vi "Source and Sink Current.vi"(0 "Semiconductor Module Context":T1, 2 "Current level":dbl=0.001 caption="current level" format="%_6p", 5 "Pins":string[](array[string]), 11 "error in (no error)":errorcluster) -> (4 "Semiconductor Module Context Out":T1, 6 "Source Current measurements":dbl[](array[numeric]), 8 "Sink Current measurements":dbl[](array[numeric]), 15 "error out":errorcluster)   [LabVIEW 2013]
uses:
  <vilib>/NI_TestStand_SemiconductorModule/NI_TestStand_Semiconductor_Module.lvlibp/PinMap/General/SemiconductorModuleContext.ctl
  <vilib>/NI_TestStand_SemiconductorModule/NI_TestStand_Semiconductor_Module.lvlibp
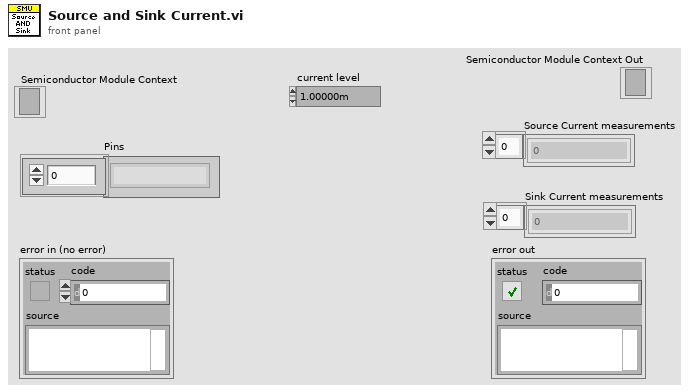
[diagram p1: front panel]
types:
  T1 = typedef "NI_TestStand_Semiconductor_Module.lvlibp/SemiconductorModuleContext.ctl" = refnum<k7>
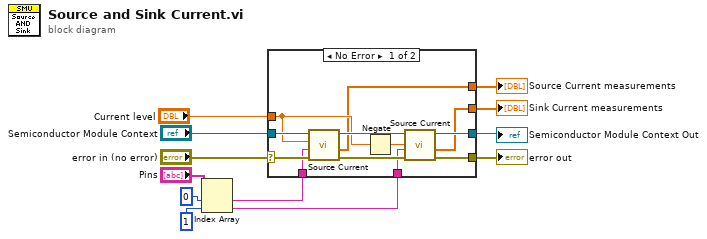
[diagram p0: block diagram]
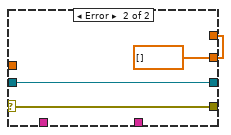
[diagram p2: hidden frame]
diagram:
  n1 = Index Array(array="Pins", index #1=0 ("index"), index #2=1 ("index")) -> (element #1=w6:string, element #2=w5:string)
  n2 = case shown="No Error" "error in (no error)" {
    selector: "error in (no error)" -> [w24 w27]
    tunnel: [w21 w27] -> w9
    tunnel: "Current level" -> [w18 _]
    tunnel: [w16 w25] -> w11
    tunnel: "Semiconductor Module Context" -> [w23 w26]
    tunnel: [w17 w26] -> w10
    tunnel: w6 -> [w15 _]
    tunnel: w5 -> [w14 _]
    tunnel: [w13 w25] -> w4
    frame No Error {
      n3 = call "Source Current.vi"("error in (no error)"=w24, "Pin"=w15, "Current level"=w18, "Semiconductor Module Context"=w23) -> ("error out"=w22:errorcluster, "current measurements"=w13:dbl[], "Semiconductor Module Context Out"=w20:T1)  [unwired: 4 in, 1 out]
      n4 = Negate(x=w18) -> (-x=w19:dbl)
      n5 = call "Source Current.vi"("error in (no error)"=w22, "Pin"=w14, "Current level"=w19, "Semiconductor Module Context"=w20) -> ("error out"=w21:errorcluster, "current measurements"=w16:dbl[], "Semiconductor Module Context Out"=w17:T1)  [unwired: 4 in, 1 out]
    }
    frame Error {
      w25 = dbl[] [] ("voltage measurements")
    }
  }
  "error out" <- w9
  "Source Current measurements" <- w4
  "Sink Current measurements" <- w11
  "Semiconductor Module Context Out" <- w10
